vi "ComputePeriodsLoop.vi"() -> ()   [LabVIEW 2019]
uses:
  <vilib>/rvi/Emulation/niFpgaGetClockAttributes.vi
  <vilib>/rvi/Emulation/niFpgaSctlEmulationGetInTimedLoop.vi
  <vilib>/rvi/Emulation/niFpgaEmulationReportErrorSimple.vi
  <vilib>/rvi/eio/common/nirviEmuTemplateMethod_errors.vi
  <vilib>/rvi/Emulation/niFpgaCriticalErrorInLSC.vi
  <vilib>/eio/EIONode/EIONode.xnode
panel:
  out "x-y 3":u32
  out "x-y 2":u32
  out "x-y":u32
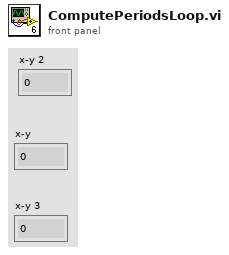
[diagram p1: front panel]
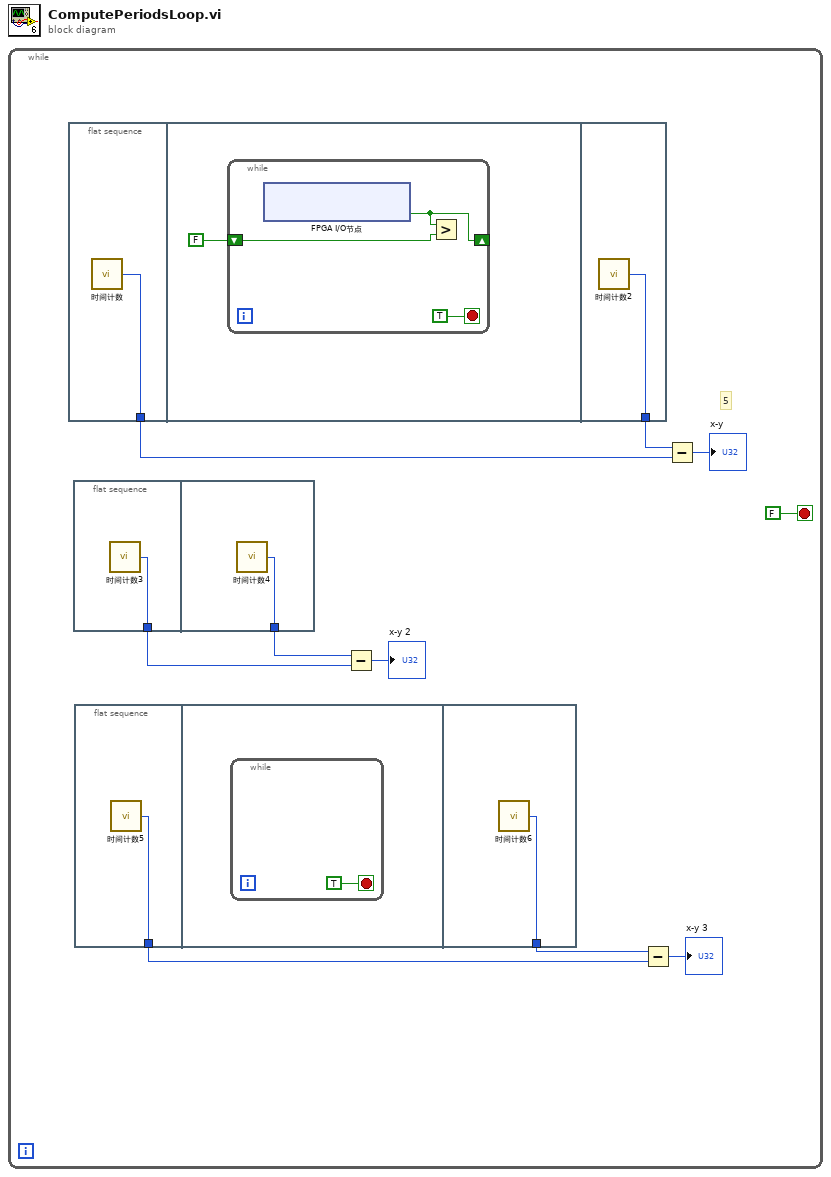
[diagram p0: block diagram]
diagram:
  n1 = while {
    stop <- FALSE stop-if-true
    # "5"
    n2 = flat-sequence {
      tunnel: [w16] -> w8
      tunnel: [w21] -> w9
      frame #0 {
        n3 = call "时间计数"() -> ("Tick Count(Ticks)"=w16:u32)
      }
      frame #1 {
        n4 = while {
          shift-right: [w19] -> _
          shift-left: FALSE -> [w20]
          stop <- TRUE stop-if-true
          n5 = xnode "FPGA I/O节点"() -> ("ConnectorB/DIO0"=w19:bool)  [unwired: 1 in, 1 out]
          n6 = Greater?(x=w19, y=w20) -> ()  [unwired: 1 out]
        }
      }
      frame #2 {
        n7 = call "时间计数2"() -> ("Tick Count(Ticks)"=w21:u32)
      }
    }
    n8 = flat-sequence {
      tunnel: [w14] -> w6
      tunnel: [w15] -> w5
      frame #0 {
        n9 = call "时间计数3"() -> ("Tick Count(Ticks)"=w14:u32)
      }
      frame #1 {
        n10 = call "时间计数4"() -> ("Tick Count(Ticks)"=w15:u32)
      }
    }
    n11 = flat-sequence {
      tunnel: [w11] -> w3
      tunnel: [w13] -> w2
      frame #0 {
        n12 = call "时间计数5"() -> ("Tick Count(Ticks)"=w11:u32)
      }
      frame #1 {
        n13 = while {
          stop <- TRUE stop-if-true
        }
      }
      frame #2 {
        n14 = call "时间计数6"() -> ("Tick Count(Ticks)"=w13:u32)
      }
    }
    n15 = Subtract(x=w5, y=w6) -> (x-y=→"x-y 2":u32)
    n16 = Subtract(x=w2, y=w3) -> (x-y=→"x-y 3":u32)
    n17 = Subtract(x=w9, y=w8) -> (x-y=→"x-y":u32)
  }
